vi "Check_If_any_condition_has_became_FALSE.vi"(2 "Error In":errorcluster, 3 "Conditions met in":bool[](array[boolean]), 4 "Reset?":bool) -> (0 "Error Out":errorcluster, 1 "Conditions became FALSE":bool[](array[boolean]))   [LabVIEW 2018, in "TTL IO.lvlib"]
uses:
  TTL IO.lvlib
  <vilib>/ptbypt/NI_PtbyPt.lvlib
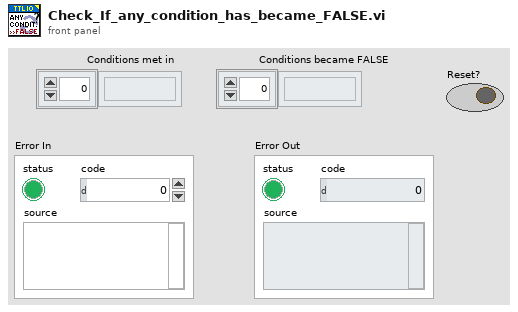
[diagram p1: front panel]
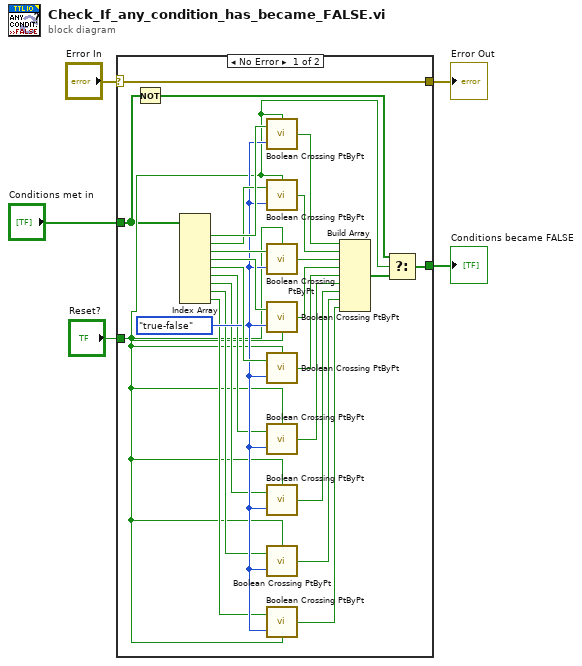
[diagram p0: block diagram]
diagram:
  n1 = case shown="No Error" "Error In" {
    selector: "Error In" -> [w30 w31]
    tunnel: [w10 _] -> w2
    tunnel: "Conditions met in" -> [w7 _]
    tunnel: [w30 w31] -> w4
    tunnel: "Reset?" -> [w8 _]
    frame No Error {
      w19 = enum16{"either", "false-true", "true-false"}."true-false" ("direction")
      n2 = Not(x=w7) -> (.not. x?=w6:bool[])
      n3 = Index Array(array=w7) -> (element #1=w29:bool, element #2=w28:bool, element #3=w27:bool, element #4=w26:bool, element #5=w21:bool, element #6=w14:bool, element #7=w13:bool, element #8=w12:bool, element #9=w11:bool)  [unwired: 9 in]
      n4 = call <vilib>:"Boolean Crossing PtByPt.vi"("initialize"=w8, "direction"=w19, "input"=w29) -> ("crossing"=w25:bool)
      n5 = call <vilib>:"Boolean Crossing PtByPt.vi"("initialize"=w8, "direction"=w19, "input"=w28) -> ("crossing"=w24:bool)
      n6 = call <vilib>:"Boolean Crossing PtByPt.vi"("initialize"=w8, "direction"=w19, "input"=w27) -> ("crossing"=w23:bool)
      n7 = call <vilib>:"Boolean Crossing PtByPt.vi"("initialize"=w8, "direction"=w19, "input"=w26) -> ("crossing"=w22:bool)
      n8 = call <vilib>:"Boolean Crossing PtByPt.vi"("initialize"=w8, "direction"=w19, "input"=w21) -> ("crossing"=w20:bool)
      n9 = call <vilib>:"Boolean Crossing PtByPt.vi"("initialize"=w8, "direction"=w19, "input"=w14) -> ("crossing"=w18:bool)
      n10 = call <vilib>:"Boolean Crossing PtByPt.vi"("initialize"=w8, "direction"=w19, "input"=w13) -> ("crossing"=w17:bool)
      n11 = call <vilib>:"Boolean Crossing PtByPt.vi"("initialize"=w8, "direction"=w19, "input"=w12) -> ("crossing"=w16:bool)
      n12 = call <vilib>:"Boolean Crossing PtByPt.vi"("initialize"=w8, "direction"=w19, "input"=w11) -> ("crossing"=w15:bool)
      n13 = Build Array(w25, w24, w23, w22, w20, w18, w17, w16, w15) -> (w9:bool[])
      n14 = Select(t=w6, s=w8, f=w9) -> (s? t:f=w10:bool[])
    }
    frame Error {
    }
  }
  "Conditions became FALSE" <- w2
  "Error Out" <- w4
